vi "模式删除节点.vi"(10 "名字":string, 11 "模式":T1) -> (2 "模式合法":bool, 3 "模式-output":T1)   [LabVIEW 2019]
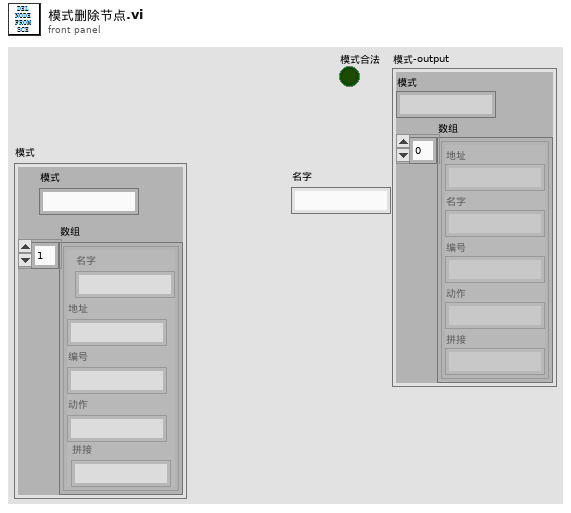
[diagram p1: front panel]
types:
  T1 = cluster{"模式":string, "数组":cluster{"地址":string, "名字":string, "编号":string, "动作":string, "拼接":string}[]}
  T2 = cluster{"地址":string, "名字":string, "编号":string, "动作":string, "拼接":string}[]
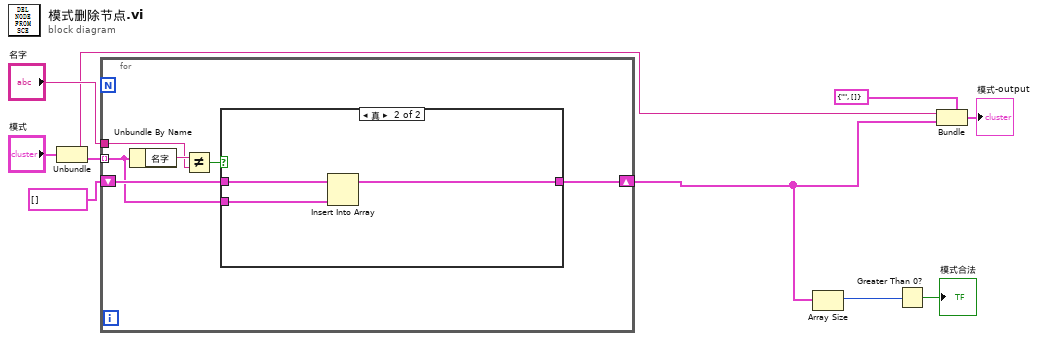
[diagram p0: block diagram]
diagram:
  n1 = Unbundle("模式") -> ("模式"=w3:string, "数组"=w9:T2)
  n2 = for {
    tunnel: w9 -> [w14] mode=indexing
    shift-right: [w16] -> w2
    shift-left: T2 [] -> [w15]
    tunnel: "名字" -> [w12]
    n3 = Unbundle By Name(w14) -> ("名字"=w13:string)
    n4 = Not Equal?(x=w13, y=w12) -> (x != y?=w11:bool)
    n5 = case shown="真" w11 {
      tunnel: [w17 w20] -> w16
      tunnel: w15 -> [w17 w19]
      tunnel: w14 -> [_ w18]
      frame False {
      }
      frame True {
        n6 = Insert Into Array(array=w19, new element=w18) -> (w20:T2)  [unwired: 1 in]
      }
    }
  }
  n7 = Array Size(array=w2) -> (size(s)=w6:i32)
  n8 = Greater Than 0?(x=w6) -> (x > 0?=→"模式合法":bool)
  n9 = Bundle(cluster=T1 {"模式"="", "数组"=[]} ("模式"), "模式"=w3, "数组"=w2) -> (→"模式-output":T1)
